vi "SCMP CoMP-S Mechanism - rotation.vi"(8 "error in (no error)":errorcluster, 9 "Auto Motors":bool, 10 "Actual Rotation":dbl, 11 "New Rotation":dbl) -> (0 "error out":errorcluster)   [LabVIEW 2014]
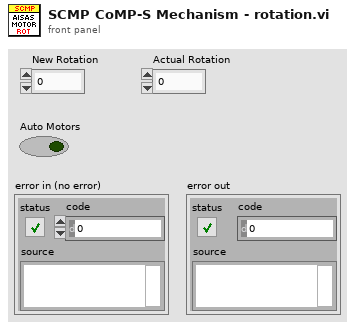
[diagram p1: front panel]
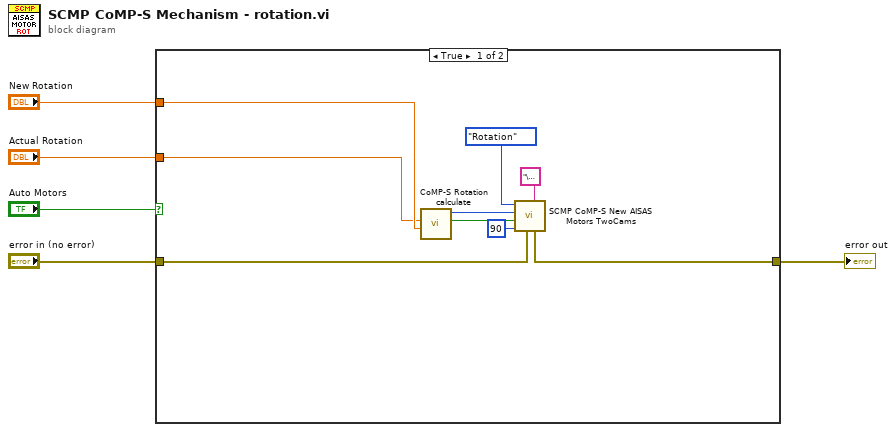
[diagram p0: block diagram]
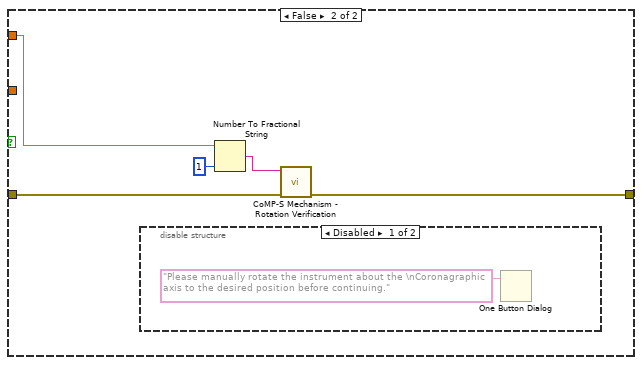
[diagram p2: hidden frame]
diagram:
  n1 = case shown="True" "Auto Motors" {
    tunnel: "error in (no error)" -> [w7 w19]
    tunnel: [w6 w18] -> w3
    tunnel: "New Rotation" -> [w10 w15]
    tunnel: "Actual Rotation" -> [w9 _]
    frame True {
      n2 = call "CoMP-S Rotation calculate.vi"("New Value"=w10, "Old Value"=w9) -> ("Direction"=w12:bool, "steps"=w11:i32)  [unwired: 6 in, 2 out]
      n3 = call "SCMP CoMP-S New AISAS Motors TwoCams.vi"("Motion Code"="\u0002", "error in (no error)"=w7, "steps/sec"=u32 90, "motor rotation"=w12, "Steps"=w11, "Motor selection"=enum32{"Rotation", "Difuser ", "Objective Lens"}."Rotation") -> ("error out"=w6:errorcluster)  [unwired: 2 in, 3 out]
    }
    frame False {
      n4 = disable-structure shown="Disabled" {
        frame Disabled {
          n5 = One Button Dialog(message="Please manually rotate the instrument about the \nCoronagraphic axis to the desired position before continuing.") -> ()  [unwired: 1 in, 1 out]
        }
        frame Enabled {
        }
      }
      n6 = Number To Fractional String(number=w15, precision (6)=i16 1) -> (F-format string=w16:string)  [unwired: 2 in]
      n7 = call "CoMP-S Mechanism - Rotation Verification.vi"("error in (no error)"=w19, "String"=w16) -> ("error out"=w18:errorcluster)  [unwired: 9 in]
    }
  }
  "error out" <- w3
